vi "Test_waitForCompletion_enterControl.vi"(8 "error in (no error)":errorcluster, 11 "waitComplete_Ctl":T1) -> (0 "error out":errorcluster, 2 "function return":i32, 3 "waitComplete_Ctl out":T1)   [LabVIEW 2018, in "SALLV_Test.lvlib"]
doc: "int Test_shm_waitForCompletion_enterControlLV(Test_waitCompleteLV *waitComplete_Ctl);"
uses:
  SALLV_Test.lvlib
  SALLV_Test.so
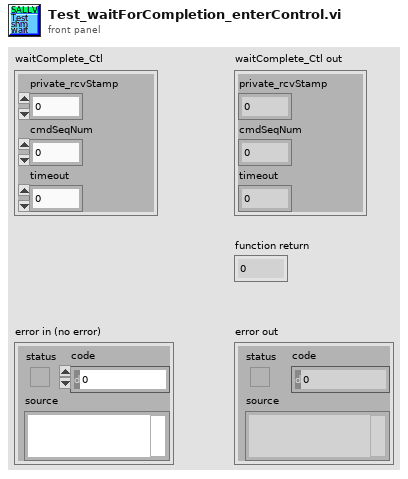
[diagram p1: front panel]
types:
  T1 = cluster{"private_rcvStamp":dbl, "cmdSeqNum":i32, "timeout":u32}
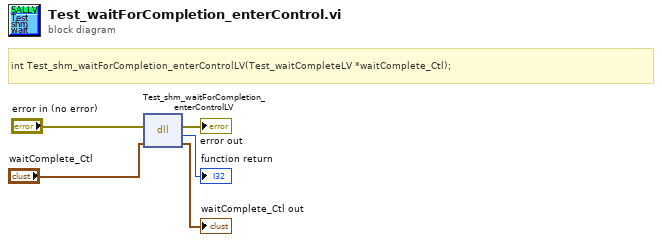
[diagram p0: block diagram]
diagram:
  # "int Test_shm_waitForCompletion_enterControlLV(Test_waitCompleteLV *waitComplete_Ctl);"
  n1 = dll-call lib="home/ttsai/Documents/salTestLabViewApi/SALLV_Test/SALLV_Test.*" fn="Test_shm_waitForCompletion_enterControlLV"(error in="error in (no error)", "waitComplete_Ctl"="waitComplete_Ctl") -> (error out=→"error out":errorcluster, →"function return":i32, "waitComplete_Ctl"=→"waitComplete_Ctl out":T1)  [unwired: 2 in, 1 out]
